vi "Load Instrument Classes.vi"(8 "error in (no error)":errorcluster, 11 "Control Experiment.lvclass":refnum<class "Control Experiment SM.lvclass">) -> (0 "error out":errorcluster, 3 "Control Experiment out":refnum<class "Control Experiment SM.lvclass">)   [LabVIEW 2016, in "Control Experiment SM.lvclass"]
uses:
  Control Experiment SM/Control Experiment SM.lvclass
  Control Experiment SM/Control Experiment SM.lvclass/Control Experiment SM.ctl
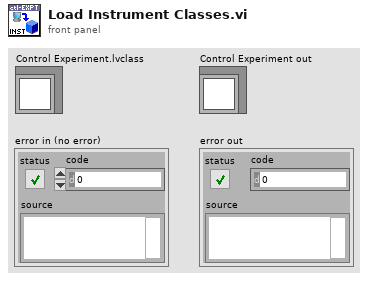
[diagram p1: front panel]
types:
  T1 = typedef "Control Experiment SM.lvclass/Instrument--enum.ctl" = enum16{"----- AFM/EBL -----", "AGILENT", "CYPHER", "Gemini2", "JEOL", "MFP3D", "----- Cryostat -----", "CF900", "DR200", "MNK", "PPMS 1", "PPMS 2", "PPMS 3", "----- Optics -----", "THz 1", "THz 2"}
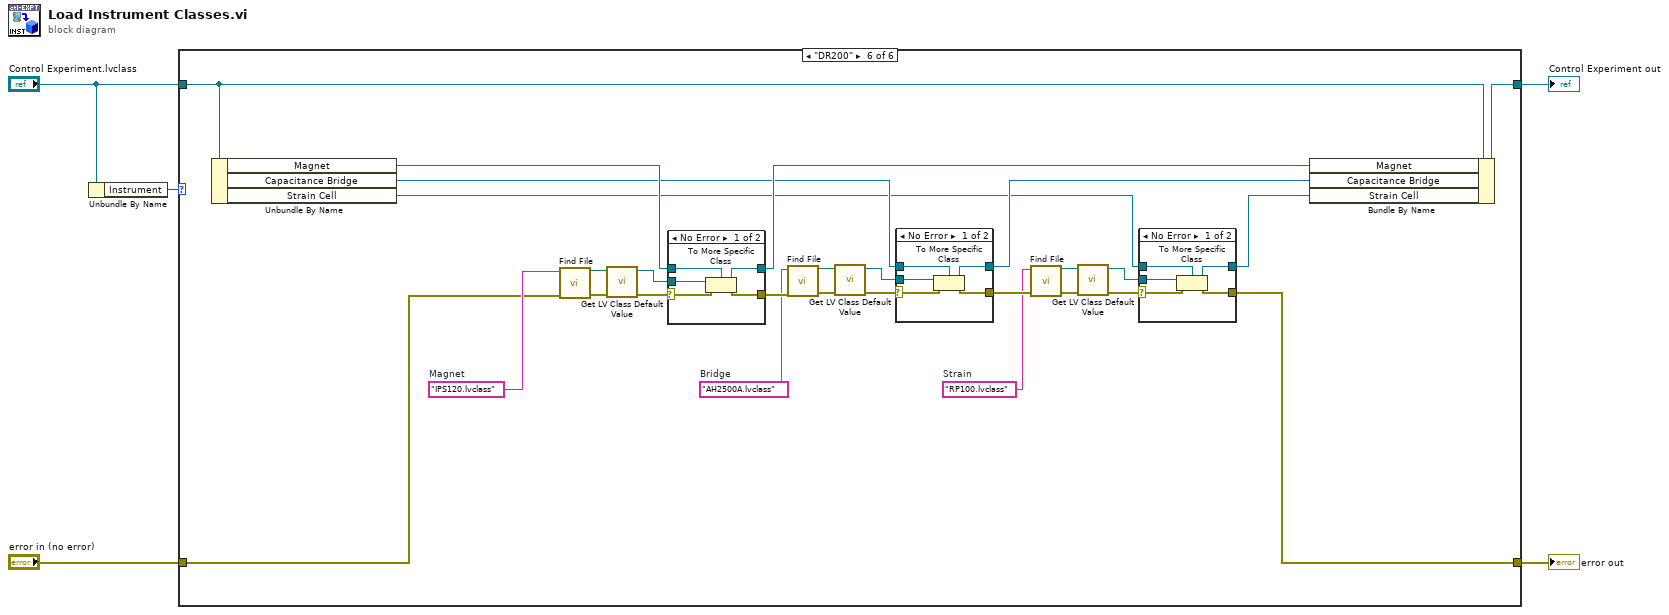
[diagram p0: block diagram]
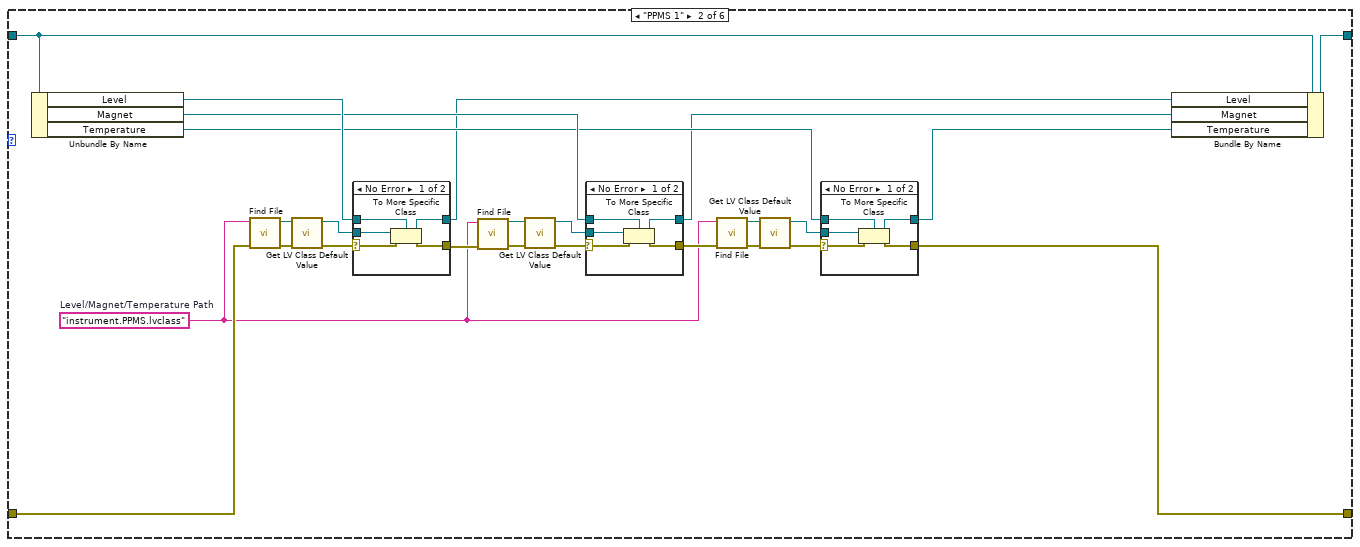
[diagram p3: hidden frame]
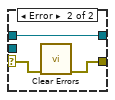
[diagram p4: hidden frame]
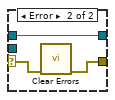
[diagram p5: hidden frame]
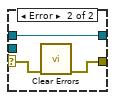
[diagram p6: hidden frame]
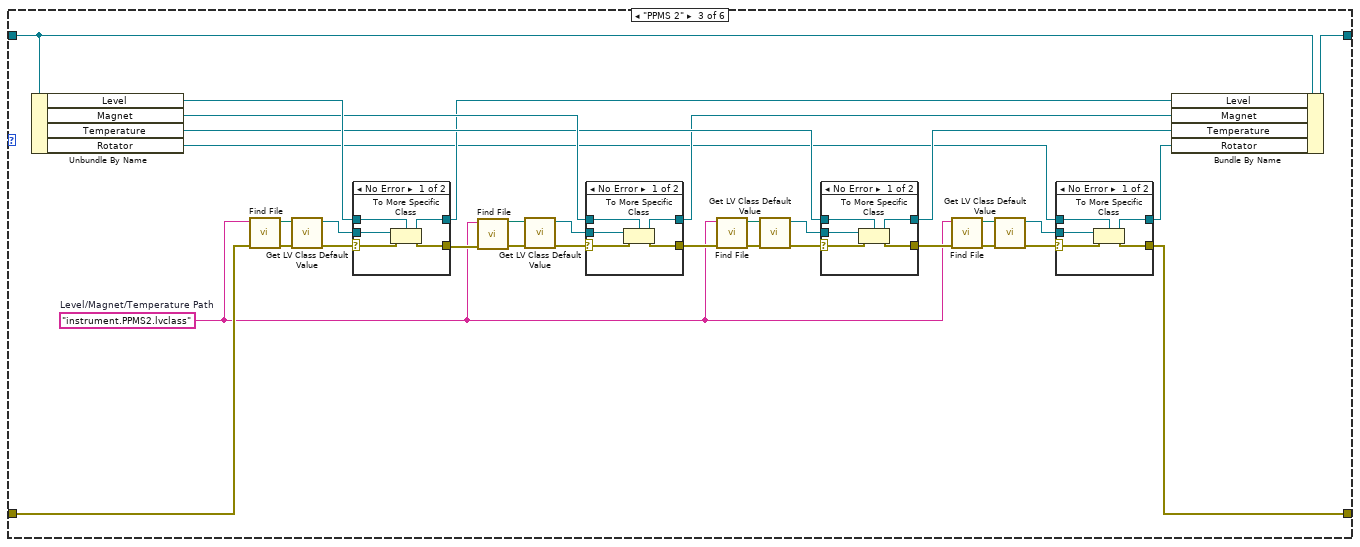
[diagram p7: hidden frame]
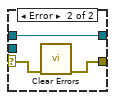
[diagram p8: hidden frame]
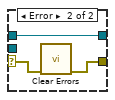
[diagram p9: hidden frame]
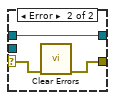
[diagram p10: hidden frame]
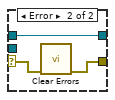
[diagram p11: hidden frame]
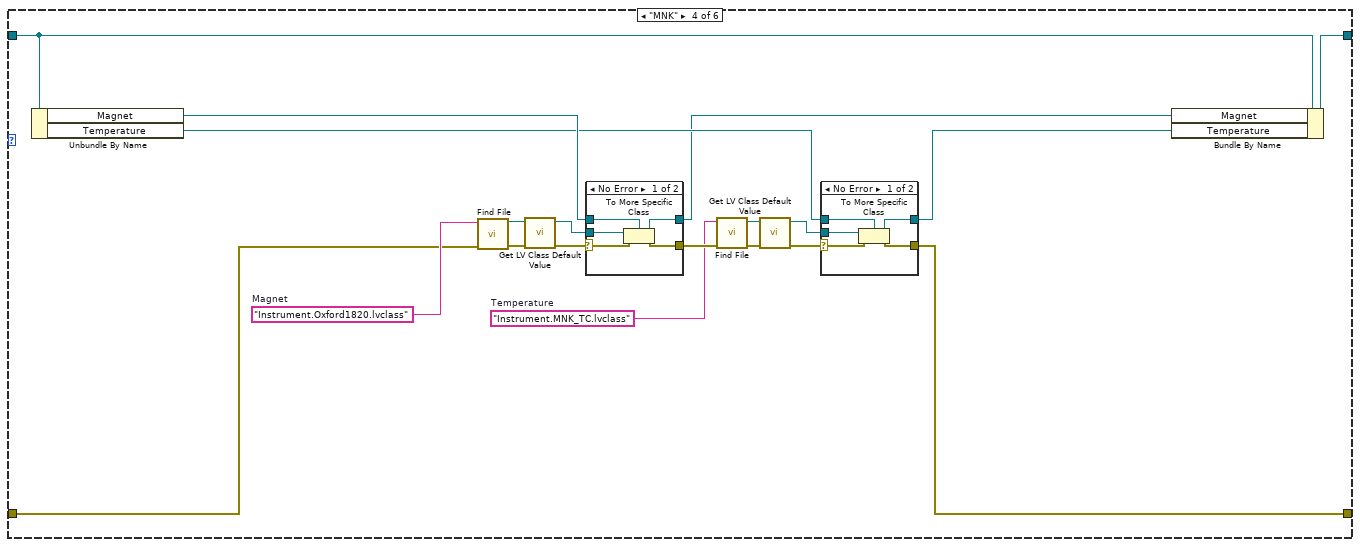
[diagram p12: hidden frame]
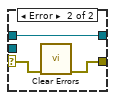
[diagram p13: hidden frame]
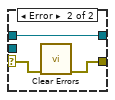
[diagram p14: hidden frame]
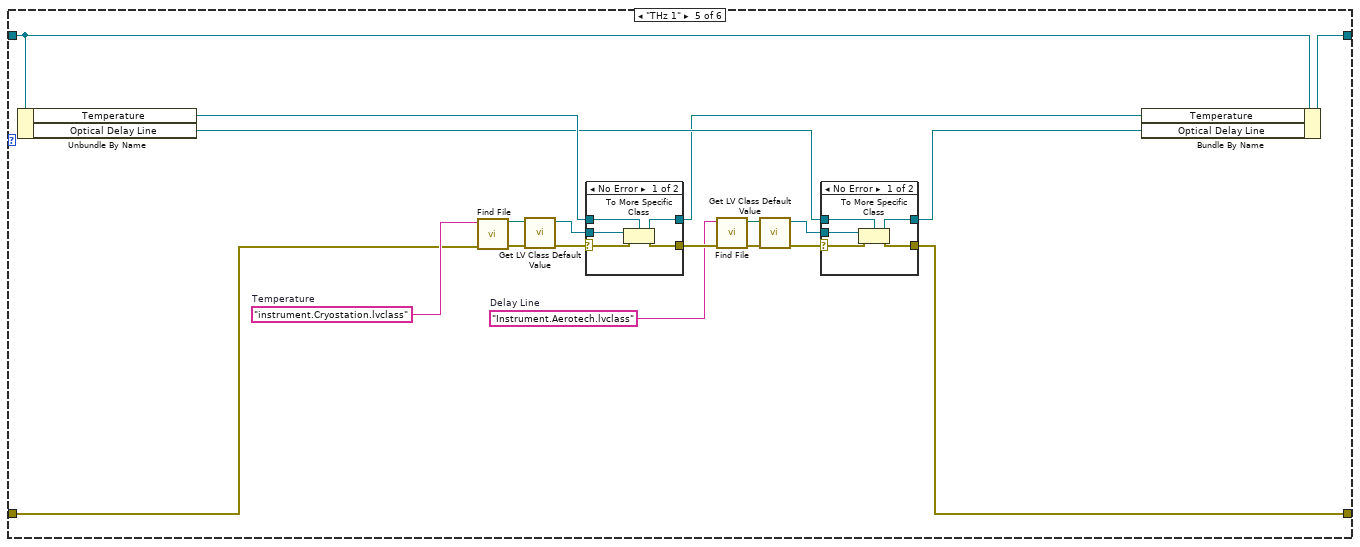
[diagram p15: hidden frame]
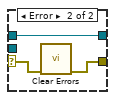
[diagram p16: hidden frame]
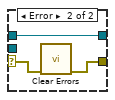
[diagram p17: hidden frame]
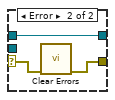
[diagram p18: hidden frame]
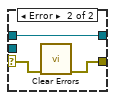
[diagram p19: hidden frame]
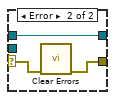
[diagram p20: hidden frame]
diagram:
  n1 = Unbundle By Name("Control Experiment.lvclass") -> ("Instrument"=w2:T1)
  n2 = case shown="\"DR200\"" w2 {
    tunnel: [w6 w18 w58 w121 w156 w191] -> w5
    tunnel: [w7 w32 w88 w139 w174 w217] -> w4
    tunnel: "Control Experiment.lvclass" -> [w7 w31 w87 w138 w173 w216]
    tunnel: "error in (no error)" -> [w6 w17 w74 w122 w157 w208]
    frame Default {
    }
    frame "PPMS 1" {
      w8 = "instrument.PPMS.lvclass"  # Level/Magnet/Temperature Path
      n3 = Unbundle By Name(w31) -> ("Level"=w28:refnum<class "Instrument.Cryostat.lvclass">, "Magnet"=w23:refnum<class "Instrument.Cryostat.lvclass">, "Temperature"=w22:refnum<class "Instrument.Cryostat.lvclass">)
      n4 = call "Find File.vi"("error in (no error)"=w17, "File Name"=w8) -> ("error out"=w19:errorcluster, "Path"=w15:path)  [unwired: 8 in]
      n5 = call <vilib>:"Get LV Class Default Value.vi"("error in (no error)"=w19, "class path"=w15) -> ("error out"=w29:errorcluster, "object"=w30:refnum<class>)  [unwired: 8 in]
      n6 = case shown="No Error" w29 {
        selector: w29 -> [w43 w46]
        tunnel: [w41 w47] -> w16
        tunnel: w30 -> [w45 _]
        tunnel: [w44 w48] -> w12
        tunnel: w28 -> [w42 w47]
        frame No Error {
          n7 = To More Specific Class(target class=w42, reference=w45, error in=w43) -> (specific class reference=w41:refnum<class "Instrument.Cryostat.lvclass">, error out=w44:errorcluster)
        }
        frame Error {
          n8 = call <vilib>:"Clear Errors.vi"("error in (no error)"=w46) -> ("error out"=w48:errorcluster)  [unwired: 5 in, 1 out]
        }
      }
      n9 = call "Find File.vi"("error in (no error)"=w12, "File Name"=w8) -> ("error out"=w14:errorcluster, "Path"=w13:path)  [unwired: 8 in]
      n10 = call <vilib>:"Get LV Class Default Value.vi"("error in (no error)"=w14, "class path"=w13) -> ("error out"=w27:errorcluster, "object"=w26:refnum<class>)  [unwired: 8 in]
      n11 = case shown="No Error" w27 {
        selector: w27 -> [w35 w38]
        tunnel: [w33 w39] -> w20
        tunnel: w26 -> [w37 _]
        tunnel: [w36 w40] -> w9
        tunnel: w23 -> [w34 w39]
        frame No Error {
          n12 = To More Specific Class(target class=w34, reference=w37, error in=w35) -> (specific class reference=w33:refnum<class "Instrument.Cryostat.lvclass">, error out=w36:errorcluster)
        }
        frame Error {
          n13 = call <vilib>:"Clear Errors.vi"("error in (no error)"=w38) -> ("error out"=w40:errorcluster)  [unwired: 5 in, 1 out]
        }
      }
      n14 = call "Find File.vi"("error in (no error)"=w9, "File Name"=w8) -> ("error out"=w11:errorcluster, "Path"=w10:path)  [unwired: 8 in]
      n15 = call <vilib>:"Get LV Class Default Value.vi"("error in (no error)"=w11, "class path"=w10) -> ("error out"=w24:errorcluster, "object"=w25:refnum<class>)  [unwired: 8 in]
      n16 = case shown="No Error" w24 {
        selector: w24 -> [w51 w54]
        tunnel: [w49 w55] -> w21
        tunnel: w25 -> [w53 _]
        tunnel: [w52 w56] -> w18
        tunnel: w22 -> [w50 w55]
        frame No Error {
          n17 = To More Specific Class(target class=w50, reference=w53, error in=w51) -> (specific class reference=w49:refnum<class "Instrument.Cryostat.lvclass">, error out=w52:errorcluster)
        }
        frame Error {
          n18 = call <vilib>:"Clear Errors.vi"("error in (no error)"=w54) -> ("error out"=w56:errorcluster)  [unwired: 5 in, 1 out]
        }
      }
      n19 = Bundle By Name(cluster=w31, "Level"=w16, "Magnet"=w20, "Temperature"=w21) -> (w32:refnum<class "Control Experiment SM.lvclass">)
    }
    frame "PPMS 2" {
      w57 = "instrument.PPMS2.lvclass"  # Level/Magnet/Temperature Path
      n20 = Unbundle By Name(w87) -> ("Level"=w84:refnum<class "Instrument.Cryostat.lvclass">, "Magnet"=w79:refnum<class "Instrument.Cryostat.lvclass">, "Temperature"=w78:refnum<class "Instrument.Cryostat.lvclass">, "Rotator"=w60:refnum<class "Instrument.Cryostat.lvclass">)
      n21 = call "Find File.vi"("error in (no error)"=w74, "File Name"=w57) -> ("error out"=w75:errorcluster, "Path"=w72:path)  [unwired: 8 in]
      n22 = call <vilib>:"Get LV Class Default Value.vi"("error in (no error)"=w75, "class path"=w72) -> ("error out"=w85:errorcluster, "object"=w86:refnum<class>)  [unwired: 8 in]
      n23 = case shown="No Error" w85 {
        selector: w85 -> [w107 w110]
        tunnel: [w105 w111] -> w73
        tunnel: w86 -> [w109 _]
        tunnel: [w108 w112] -> w69
        tunnel: w84 -> [w106 w111]
        frame No Error {
          n24 = To More Specific Class(target class=w106, reference=w109, error in=w107) -> (specific class reference=w105:refnum<class "Instrument.Cryostat.lvclass">, error out=w108:errorcluster)
        }
        frame Error {
          n25 = call <vilib>:"Clear Errors.vi"("error in (no error)"=w110) -> ("error out"=w112:errorcluster)  [unwired: 5 in, 1 out]
        }
      }
      n26 = call "Find File.vi"("error in (no error)"=w69, "File Name"=w57) -> ("error out"=w71:errorcluster, "Path"=w70:path)  [unwired: 8 in]
      n27 = call <vilib>:"Get LV Class Default Value.vi"("error in (no error)"=w71, "class path"=w70) -> ("error out"=w83:errorcluster, "object"=w82:refnum<class>)  [unwired: 8 in]
      n28 = case shown="No Error" w83 {
        selector: w83 -> [w99 w102]
        tunnel: [w97 w103] -> w76
        tunnel: w82 -> [w101 _]
        tunnel: [w100 w104] -> w66
        tunnel: w79 -> [w98 w103]
        frame No Error {
          n29 = To More Specific Class(target class=w98, reference=w101, error in=w99) -> (specific class reference=w97:refnum<class "Instrument.Cryostat.lvclass">, error out=w100:errorcluster)
        }
        frame Error {
          n30 = call <vilib>:"Clear Errors.vi"("error in (no error)"=w102) -> ("error out"=w104:errorcluster)  [unwired: 5 in, 1 out]
        }
      }
      n31 = call "Find File.vi"("error in (no error)"=w66, "File Name"=w57) -> ("error out"=w68:errorcluster, "Path"=w67:path)  [unwired: 8 in]
      n32 = call <vilib>:"Get LV Class Default Value.vi"("error in (no error)"=w68, "class path"=w67) -> ("error out"=w80:errorcluster, "object"=w81:refnum<class>)  [unwired: 8 in]
      n33 = case shown="No Error" w80 {
        selector: w80 -> [w115 w118]
        tunnel: [w113 w119] -> w77
        tunnel: w81 -> [w117 _]
        tunnel: [w116 w120] -> w61
        tunnel: w78 -> [w114 w119]
        frame No Error {
          n34 = To More Specific Class(target class=w114, reference=w117, error in=w115) -> (specific class reference=w113:refnum<class "Instrument.Cryostat.lvclass">, error out=w116:errorcluster)
        }
        frame Error {
          n35 = call <vilib>:"Clear Errors.vi"("error in (no error)"=w118) -> ("error out"=w120:errorcluster)  [unwired: 5 in, 1 out]
        }
      }
      n36 = call "Find File.vi"("error in (no error)"=w61, "File Name"=w57) -> ("error out"=w64:errorcluster, "Path"=w65:path)  [unwired: 8 in]
      n37 = call <vilib>:"Get LV Class Default Value.vi"("error in (no error)"=w64, "class path"=w65) -> ("error out"=w63:errorcluster, "object"=w62:refnum<class>)  [unwired: 8 in]
      n38 = case shown="No Error" w63 {
        selector: w63 -> [w91 w94]
        tunnel: [w89 w95] -> w59
        tunnel: w62 -> [w93 _]
        tunnel: [w92 w96] -> w58
        tunnel: w60 -> [w90 w95]
        frame No Error {
          n39 = To More Specific Class(target class=w90, reference=w93, error in=w91) -> (specific class reference=w89:refnum<class "Instrument.Cryostat.lvclass">, error out=w92:errorcluster)
        }
        frame Error {
          n40 = call <vilib>:"Clear Errors.vi"("error in (no error)"=w94) -> ("error out"=w96:errorcluster)  [unwired: 5 in, 1 out]
        }
      }
      n41 = Bundle By Name(cluster=w87, "Level"=w73, "Magnet"=w76, "Temperature"=w77, "Rotator"=w59) -> (w88:refnum<class "Control Experiment SM.lvclass">)
    }
    frame "MNK" {
      w124 = "Instrument.MNK_TC.lvclass"  # Temperature
      w123 = "Instrument.Oxford1820.lvclass"  # Magnet
      n42 = Unbundle By Name(w138) -> ("Magnet"=w133:refnum<class "Instrument.Cryostat.lvclass">, "Temperature"=w132:refnum<class "Instrument.Cryostat.lvclass">)
      n43 = call "Find File.vi"("error in (no error)"=w122, "File Name"=w123) -> ("error out"=w129:errorcluster, "Path"=w128:path)  [unwired: 8 in]
      n44 = call <vilib>:"Get LV Class Default Value.vi"("error in (no error)"=w129, "class path"=w128) -> ("error out"=w137:errorcluster, "object"=w136:refnum<class>)  [unwired: 8 in]
      n45 = case shown="No Error" w137 {
        selector: w137 -> [w142 w145]
        tunnel: [w140 w146] -> w130
        tunnel: w136 -> [w144 _]
        tunnel: [w143 w147] -> w125
        tunnel: w133 -> [w141 w146]
        frame No Error {
          n46 = To More Specific Class(target class=w141, reference=w144, error in=w142) -> (specific class reference=w140:refnum<class "Instrument.Cryostat.lvclass">, error out=w143:errorcluster)
        }
        frame Error {
          n47 = call <vilib>:"Clear Errors.vi"("error in (no error)"=w145) -> ("error out"=w147:errorcluster)  [unwired: 5 in, 1 out]
        }
      }
      n48 = call "Find File.vi"("error in (no error)"=w125, "File Name"=w124) -> ("error out"=w127:errorcluster, "Path"=w126:path)  [unwired: 8 in]
      n49 = call <vilib>:"Get LV Class Default Value.vi"("error in (no error)"=w127, "class path"=w126) -> ("error out"=w134:errorcluster, "object"=w135:refnum<class>)  [unwired: 8 in]
      n50 = case shown="No Error" w134 {
        selector: w134 -> [w150 w153]
        tunnel: [w148 w154] -> w131
        tunnel: w135 -> [w152 _]
        tunnel: [w151 w155] -> w121
        tunnel: w132 -> [w149 w154]
        frame No Error {
          n51 = To More Specific Class(target class=w149, reference=w152, error in=w150) -> (specific class reference=w148:refnum<class "Instrument.Cryostat.lvclass">, error out=w151:errorcluster)
        }
        frame Error {
          n52 = call <vilib>:"Clear Errors.vi"("error in (no error)"=w153) -> ("error out"=w155:errorcluster)  [unwired: 5 in, 1 out]
        }
      }
      n53 = Bundle By Name(cluster=w138, "Magnet"=w130, "Temperature"=w131) -> (w139:refnum<class "Control Experiment SM.lvclass">)
    }
    frame "THz 1" {
      w159 = "Instrument.Aerotech.lvclass"  # Delay Line
      w158 = "instrument.Cryostation.lvclass"  # Temperature
      n54 = Unbundle By Name(w173) -> ("Temperature"=w168:refnum<class "Instrument.Cryostat.lvclass">, "Optical Delay Line"=w167:refnum<class "Instrument.OpticalDelayLine.lvclass">)
      n55 = call "Find File.vi"("error in (no error)"=w157, "File Name"=w158) -> ("error out"=w164:errorcluster, "Path"=w163:path)  [unwired: 8 in]
      n56 = call <vilib>:"Get LV Class Default Value.vi"("error in (no error)"=w164, "class path"=w163) -> ("error out"=w172:errorcluster, "object"=w171:refnum<class>)  [unwired: 8 in]
      n57 = case shown="No Error" w172 {
        selector: w172 -> [w177 w180]
        tunnel: [w175 w181] -> w165
        tunnel: w171 -> [w179 _]
        tunnel: [w178 w182] -> w160
        tunnel: w168 -> [w176 w181]
        frame No Error {
          n58 = To More Specific Class(target class=w176, reference=w179, error in=w177) -> (specific class reference=w175:refnum<class "Instrument.Cryostat.lvclass">, error out=w178:errorcluster)
        }
        frame Error {
          n59 = call <vilib>:"Clear Errors.vi"("error in (no error)"=w180) -> ("error out"=w182:errorcluster)  [unwired: 5 in, 1 out]
        }
      }
      n60 = call "Find File.vi"("error in (no error)"=w160, "File Name"=w159) -> ("error out"=w162:errorcluster, "Path"=w161:path)  [unwired: 8 in]
      n61 = call <vilib>:"Get LV Class Default Value.vi"("error in (no error)"=w162, "class path"=w161) -> ("error out"=w169:errorcluster, "object"=w170:refnum<class>)  [unwired: 8 in]
      n62 = case shown="No Error" w169 {
        selector: w169 -> [w185 w188]
        tunnel: [w183 w189] -> w166
        tunnel: w170 -> [w187 _]
        tunnel: [w186 w190] -> w156
        tunnel: w167 -> [w184 w189]
        frame No Error {
          n63 = To More Specific Class(target class=w184, reference=w187, error in=w185) -> (specific class reference=w183:refnum<class "Instrument.OpticalDelayLine.lvclass">, error out=w186:errorcluster)
        }
        frame Error {
          n64 = call <vilib>:"Clear Errors.vi"("error in (no error)"=w188) -> ("error out"=w190:errorcluster)  [unwired: 5 in, 1 out]
        }
      }
      n65 = Bundle By Name(cluster=w173, "Temperature"=w165, "Optical Delay Line"=w166) -> (w174:refnum<class "Control Experiment SM.lvclass">)
    }
    frame "DR200" {
      w194 = "RP100.lvclass"  # Strain
      w202 = "AH2500A.lvclass"  # Bridge
      w209 = "IPS120.lvclass"  # Magnet
      n66 = Unbundle By Name(w216) -> ("Magnet"=w213:refnum<class "Instrument.Cryostat.lvclass">, "Capacitance Bridge"=w200:refnum<class "Instrument.CBridge.lvclass">, "Strain Cell"=w193:refnum<class "Instrument.Strain.lvclass">)
      n67 = call "Find File.vi"("error in (no error)"=w208, "File Name"=w209) -> ("error out"=w211:errorcluster, "Path"=w210:path)  [unwired: 8 in]
      n68 = call <vilib>:"Get LV Class Default Value.vi"("error in (no error)"=w211, "class path"=w210) -> ("error out"=w215:errorcluster, "object"=w214:refnum<class>)  [unwired: 8 in]
      n69 = case shown="No Error" w215 {
        selector: w215 -> [w236 w239]
        tunnel: [w234 w240] -> w212
        tunnel: w214 -> [w238 _]
        tunnel: [w237 w241] -> w203
        tunnel: w213 -> [w235 w240]
        frame No Error {
          n70 = To More Specific Class(target class=w235, reference=w238, error in=w236) -> (specific class reference=w234:refnum<class "Instrument.Cryostat.lvclass">, error out=w237:errorcluster)
        }
        frame Error {
          n71 = call <vilib>:"Clear Errors.vi"("error in (no error)"=w239) -> ("error out"=w241:errorcluster)  [unwired: 5 in, 1 out]
        }
      }
      n72 = call "Find File.vi"("error in (no error)"=w203, "File Name"=w202) -> ("error out"=w206:errorcluster, "Path"=w207:path)  [unwired: 8 in]
      n73 = call <vilib>:"Get LV Class Default Value.vi"("error in (no error)"=w206, "class path"=w207) -> ("error out"=w204:errorcluster, "object"=w205:refnum<class>)  [unwired: 8 in]
      n74 = case shown="No Error" w204 {
        selector: w204 -> [w228 w231]
        tunnel: [w226 w232] -> w201
        tunnel: w205 -> [w230 _]
        tunnel: [w229 w233] -> w195
        tunnel: w200 -> [w227 w232]
        frame No Error {
          n75 = To More Specific Class(target class=w227, reference=w230, error in=w228) -> (specific class reference=w226:refnum<class "Instrument.CBridge.lvclass">, error out=w229:errorcluster)
        }
        frame Error {
          n76 = call <vilib>:"Clear Errors.vi"("error in (no error)"=w231) -> ("error out"=w233:errorcluster)  [unwired: 5 in, 1 out]
        }
      }
      n77 = call "Find File.vi"("error in (no error)"=w195, "File Name"=w194) -> ("error out"=w197:errorcluster, "Path"=w196:path)  [unwired: 8 in]
      n78 = call <vilib>:"Get LV Class Default Value.vi"("error in (no error)"=w197, "class path"=w196) -> ("error out"=w199:errorcluster, "object"=w198:refnum<class>)  [unwired: 8 in]
      n79 = case shown="No Error" w199 {
        selector: w199 -> [w220 w223]
        tunnel: [w218 w224] -> w192
        tunnel: w198 -> [w222 _]
        tunnel: [w221 w225] -> w191
        tunnel: w193 -> [w219 w224]
        frame No Error {
          n80 = To More Specific Class(target class=w219, reference=w222, error in=w220) -> (specific class reference=w218:refnum<class "Instrument.Strain.lvclass">, error out=w221:errorcluster)
        }
        frame Error {
          n81 = call <vilib>:"Clear Errors.vi"("error in (no error)"=w223) -> ("error out"=w225:errorcluster)  [unwired: 5 in, 1 out]
        }
      }
      n82 = Bundle By Name(cluster=w216, "Magnet"=w212, "Capacitance Bridge"=w201, "Strain Cell"=w192) -> (w217:refnum<class "Control Experiment SM.lvclass">)
    }
  }
  "error out" <- w5
  "Control Experiment out" <- w4
